vi "Get New Chess Color.vi"(8 "white available position":i32, 9 "black available position":i32, 11 "current color":T1=1) -> (3 "new color":T1=2)   [LabVIEW 2011, in "Othello.xctl"]
uses:
  Othello.xctl
  Control/Pict Ring Chess.ctl
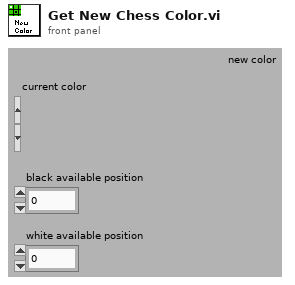
[diagram p1: front panel]
types:
  T1 = typedef "Othello.xctl/Pict Ring Chess.ctl" = u16
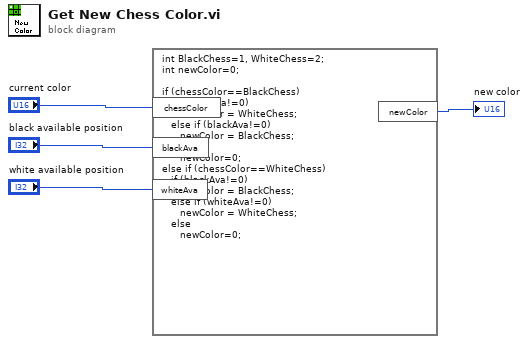
[diagram p0: block diagram]
diagram:
  n1 = formula code="int BlackChess=1, WhiteChess=2;\nint newColor=0;\n\nif (chessColor==BlackChess)\n   if (whiteAva!=0)\n      newColor = WhiteChess;\n   else if (blackAva!=0)\n      newColor = BlackChess;\n   else\n      newColor=0;\nelse if (chessColor==WhiteChess)\n   if (blackAva!=0)\n      newColor = BlackChess;\n   else if (whiteAva!=0)\n      newColor = WhiteChess;\n   else\n      newColor=0;"("chessColor"="current color", "blackAva"="black available position", "whiteAva"="white available position") -> ("newColor"=→"new color":i32)
